vi "Append To Dataset 3D Integer.vi"(8 "error in (no error)":errorcluster, 10 "data":i32[][][](array[numeric]), 11 "dataset_id":i32) -> (0 "error out":errorcluster, 3 "Dataset id out":i32)   [LabVIEW 2016]
uses:
  HDF5Tools.lvlib
  Release/HDF5Tools.dll
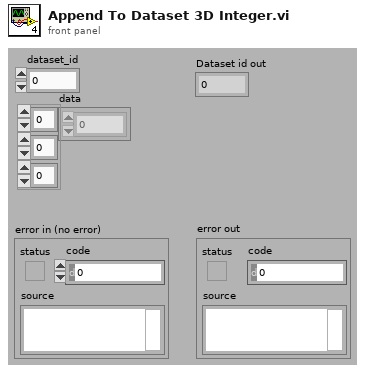
[diagram p1: front panel]
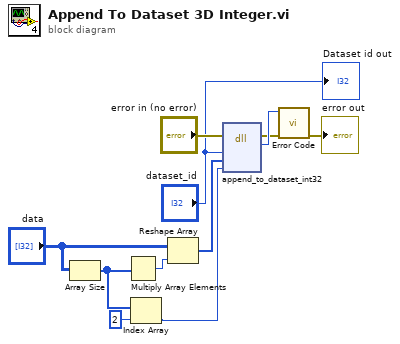
[diagram p0: block diagram]
diagram:
  n1 = Array Size(array="data") -> (size(s)=w4:i32[])
  n2 = Multiply Array Elements(1:w4) -> (0:w3:i32)
  n3 = Index Array(array=w4, index=2) -> (element=w1:i32)
  n4 = Reshape Array("data", w3) -> (w10:i32[])
  n5 = dll-call lib="Z:/users/Manolis/Labview/Cajal/private/HDF5Tools32/Release/HDF5Tools.dll" fn="append_to_dataset_int32"(error in="error in (no error)", "dataset_id"="dataset_id", "data"=w10, "count"=w1) -> (error out=w7:errorcluster, "error"=w8:i32)  [unwired: 5 in, 1 out]
  n6 = call "Error Code.vi"("Error in"=w7, "Error code"=w8) -> ("Error out"=→"error out":errorcluster)  [unwired: 9 in]
  "Dataset id out" <- "dataset_id"
